vi "Close Transport.vi"(8 "error in (no error)":errorcluster, 11 "QueueTransport":refnum<class "QueueTransport.lvclass">) -> (0 "error out":errorcluster)   [LabVIEW 2017, in "QueueTransport.lvclass"]
uses:
  QueueTransport.lvclass
  QueueTransport.lvclass/QueueTransport.ctl
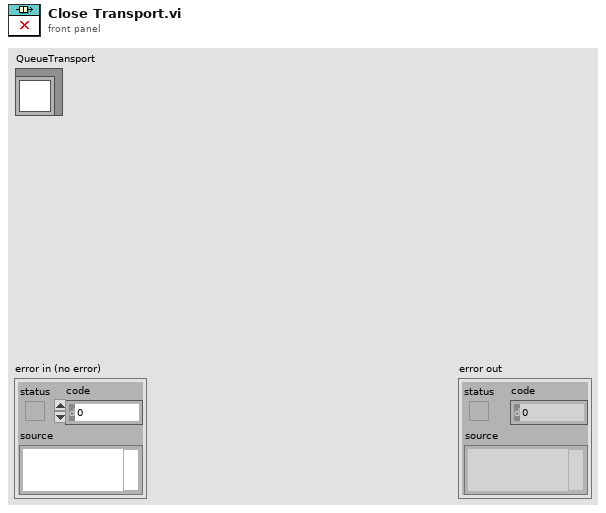
[diagram p1: front panel]
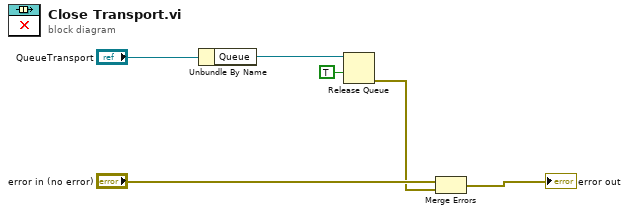
[diagram p0: block diagram]
diagram:
  n1 = Unbundle By Name("QueueTransport") -> ("Queue"=w3:refnum<queue>)
  n2 = Release Queue(queue=w3, force destroy? (F)=TRUE) -> (error out=w1:errorcluster)  [unwired: 1 in, 2 out]
  n3 = Merge Errors("error in (no error)", w1) -> (→"error out":errorcluster)
